vi "AGILENT34401a_read.vi"(0 "VISA Resource Name in":refnum<visa-resource-name>="GPIB0::22::INSTR") -> (1 "VISA Resource Name out":refnum<visa-resource-name>="GPIB0::22::INSTR", 2 "Voltage output":dbl=-0.056988192, 3 "error out":errorcluster)   [LabVIEW 2011]
panel:
  in  "Command":string="INIT\nFETC?"
  in  "Byte count":i16=1024
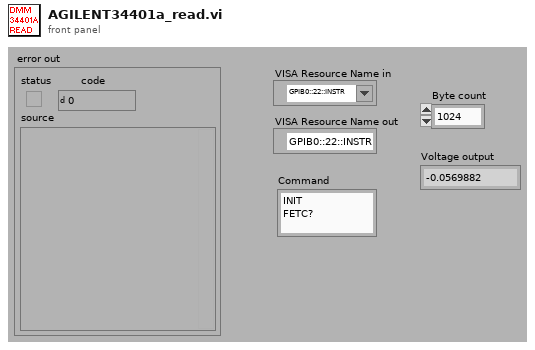
[diagram p1: front panel]
types:
  T1 = cluster{"error":bool, "code":i32, "source":string}
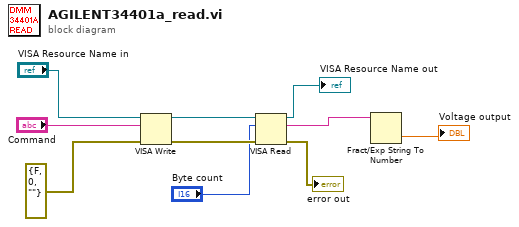
[diagram p0: block diagram]
diagram:
  n1 = VISA Write(VISA resource name="VISA Resource Name in", write buffer="Command", error in (no error)=T1 {"error"=FALSE, "code"=0, "source"=""} ("error in")) -> (VISA resource name out=w7:refnum<visa-resource-name>, error out=w6:errorcluster)  [unwired: 1 out]
  n2 = VISA Read(VISA resource name=w7, byte count="Byte count", error in (no error)=w6) -> (VISA resource name out=→"VISA Resource Name out":refnum<visa-resource-name>, read buffer=w2:string, error out=→"error out":errorcluster)  [unwired: 1 out]
  n3 = Fract/Exp String To Number(string=w2) -> (number=→"Voltage output":dbl)  [unwired: 4 out]
